vi "FTW-Tag-GetVariant.vi"(0 "FTW Actor Connector In":refnum<class "FTW-ActorConnector.lvclass">, 5 "Tag Object":variant, 11 "error in (no error)":errorcluster) -> (4 "FTW Actor Connector":refnum<class "FTW-ActorConnector.lvclass">, 6 "Response":string, 14 "Roundtrip Time":dbl format="%.6f sec", 15 "error out":errorcluster)   [LabVIEW 2015]
uses:
  Connector/FTW-ActorConnector.lvclass
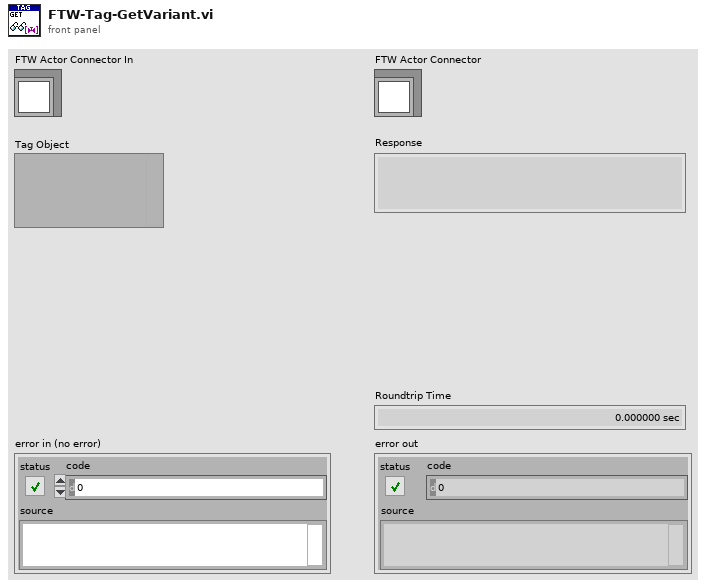
[diagram p1: front panel]
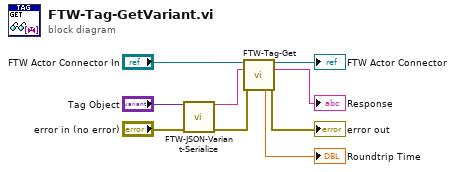
[diagram p0: block diagram]
diagram:
  n1 = call "FTW-JSON-Variant-Serialize.vi"("Variant"="Tag Object", "error in"="error in (no error)") -> ("JSON String"=w1:string, "error out"=w3:errorcluster)  [unwired: 12 in]
  n2 = call "FTW-Tag-Get.vi"("FTW Actor Connector In"="FTW Actor Connector In", "Tag Object"=w1, "error in (no error)"=w3) -> ("FTW Actor Connector"=→"FTW Actor Connector":refnum<class "FTW-ActorConnector.lvclass">, "Response"=→"Response":string, "Roundtrip Time"=→"Roundtrip Time":dbl, "error out"=→"error out":errorcluster)  [unwired: 9 in]
